vi "New .NET Drawer.vi"(7 "TextRenderingHint":i32(ring)=4 items=["SystemDefault", "SingleBitPerPixelGridFit", "SingleBitPerPixel", "AntiAliasGridFit", "AntiAlias", "ClearTypeGridFit"], 8 "error in (no error)":errorcluster, 11 "Size":cluster{"width":i32, "height":i32}={"width"=128, "height"=128}) -> (0 "error out":errorcluster, 3 "Canvas out":refnum<class "Drawer .Net.lvclass">)   [LabVIEW 2023, in "Glyph .NET Drawer.lvlib" / "Drawer .Net.lvclass"]
uses:
  Drawer .Net.lvclass
  Drawer .Net.lvclass/Drawer .Net.ctl
  System.Drawing
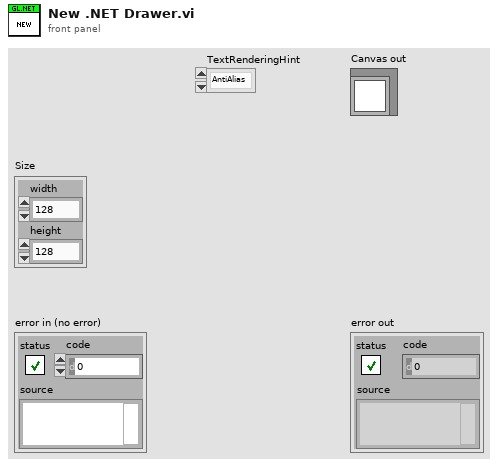
[diagram p1: front panel]
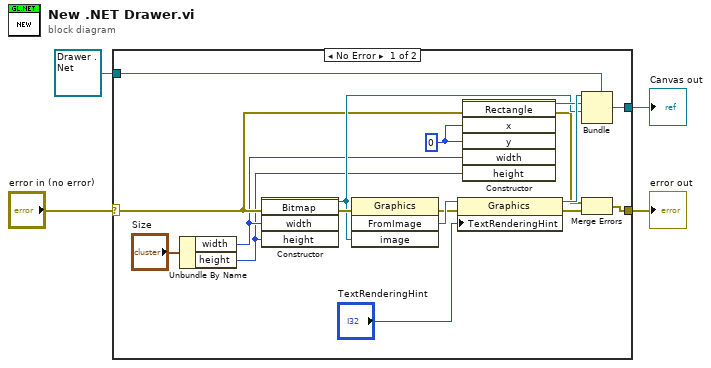
[diagram p0: block diagram]
diagram:
  n1 = case shown="No Error" "error in (no error)" {
    selector: "error in (no error)" -> [w10 w23]
    tunnel: [w11 w23] -> w3
    tunnel: [w17 w22] -> w1
    tunnel: refnum<class "Drawer .Net.lvclass"> refnum ("Canvas in") -> [w21 w22]
    frame No Error {
      w19 = 0 ("x")
      n2 = Unbundle By Name("Size") -> ("width"=w6:i32, "height"=w5:i32)
      n3 = constructor class="Bitmap"(error in=w10, "width"=w6, "height"=w5) -> (reference out=w14:refnum<k24>, error out=w20:errorcluster)  [unwired: 2 in, 3 out]
      n4 = invoke class="Graphics" method="FromImage"(error in=w20, "image"=w14) -> (error out=w8:errorcluster, "FromImage"=w9:refnum<k24>)  [unwired: 2 in, 2 out]
      n5 = property class="Graphics"(reference=w9, error in=w8, "TextRenderingHint"="TextRenderingHint") -> (reference out=w16:refnum<k24>, error out=w13:errorcluster)
      n6 = constructor class="Rectangle"(error in=w10, "x"=w19, "y"=w19, "width"=w6, "height"=w5) -> (reference out=w15:refnum<k24>, error out=w12:errorcluster)  [unwired: 2 in, 5 out]
      n7 = Bundle(cluster=w21, w16, w15, w14) -> (w17:refnum<class "Drawer .Net.lvclass">)  [unwired: 1 in]
      n8 = Merge Errors(w12, w13) -> (w11:errorcluster)
    }
    frame Error {
    }
  }
  "error out" <- w3
  "Canvas out" <- w1
